vi "HEWH Find Draw Start.vi"(6 "Loop Index":i32, 7 "Index Type":T1, 8 "Error In":errorcluster, 10 "Start Index":i32, 11 "UEF Calculated Values in":T2 {"Data Indexes"."15 sec after Draw Index" format="%#.2f"; "Data Indexes"."15 sec after Draw Timestamp" format="%#.2f"; "Data Indexes"."Test Start Timestamp" format="%.2f"; "Data Indexes"."Test End Timestamp" format="%.2f"; "Data Indexes"."T0 Timestamp" format="%.2f"; "Data Indexes"."Tsf Timestamp" format="%.2f"; "Data Indexes"."Tsu0 Timestamp" format="%.2f"; "Data Indexes"."Tmax1 Timestamp" format="%.2f"; "Data Indexes"."Draw Index Timestamp" format="%#.2f"; "Data Indexes"."Non-Draw Timestamp" format="%#.2f"; "Data Indexes"."Heating Timestamp" format="%#.2f"; "Data Indexes"."Start Energy (BTU-Gas)" format="%.6f"; "Data Indexes"."Start Watt Hours" format="%.6f"; "Static Data"."V - Volume of Wh (True)" format="%.5f"; "Static Data"."T-Ambinet Nominal (°F)" format="%.5f"; "Static Data"."T-Inlet Setpoint (°F)" format="%.5f"; "Static Data"."T-Wh Setpoint (°F)" format="%.5f"; "Sampled Data"."Qe (Wh)" format="%.5f"; "Sampled Data"."Tau stby2 (hr)" format="%.5f"; "Sampled Data"."Tastby2 (°F)" format="%.5f"; "Sampled Data"."Qf (BTU)" format="%.5f"; "Sampled Data"."Qe (BTU)" format="%.5f"; "Sampled Data"."Tmax1 (°F)" format="%.5f"; "Sampled Data"."T0 (°F)" format="%.5f"; "Sampled Data"."Qr (BTU)" format="%.5f"; "Sampled Data"."T 24(°F)" format="%.5f"; "Sampled Data"."T astby(°F)" format="%.5f"; "Sampled Data"."T tstby(°F)" format="%.5f"; "Sampled Data"."T su0(°F)" format="%.5f"; "Sampled Data"."T suf(°F)" format="%.5f"; "Sampled Data"."Tau stby_1 (hr)" format="%.5f"; "Sampled Data"."Qsuf (BTU)" format="%.5f"; "Sampled Data"."Qsu0 (BTU)" format="%.5f"; "Calculated Values"."Draw Bonus Volume (gal)" format="%.6f"; "Calculated Values"."Adjustment Factor" format="%.6f"; "Calculated Values"."T*avg_del(n-1)" format="%.6f"; "Calculated Values"."T*min(n-1)" format="%.6f"; "Calculated Values"."T*avg_del(n)" format="%.6f"; "Calculated Values"."Vn" format="%.6f"; "Calculated Values"."Qdm (BTU)" format="%.6f"; "Calculated Values"."QHWD (BTU)" format="%.6f"; "Calculated Values"."QHW (BTU)" format="%.6f"; "Calculated Values"."UEF" format="%.6f"; "Calculated Values"."QHW67 (BTU)" format="%.6f"; "Calculated Values"."Qda (BTU)" format="%.6f"; "Calculated Values"."Qd (BTU)" format="%.6f"; "Calculated Values"."Q (BTU)" format="%.6f"; "Calculated Values"."UA (BTU/(hr*F))" format="%.6f"; "Calculated Values"."Qhr (BTU/hr)" format="%.6f"; "Calculated Values"."Qstby (BTU)" format="%.6f"; "Calculated Values"."nu_r" format="%.6f"; "Calculated Values"."CpUEF (BTU/(lb*F))" format="%.6f"; "Calculated Values"."rho_nu (lb/gal)" format="%.6f"; "Calculated Values"."V1- Vol (Gal)" format="%.6f"; "Calculated Values"."M cluster mass removed (lb)" format="%.6f"; "Calculated Values"."Cp theoretical (BTU/(lbm °F))" format="%.6f"; "Calculated Values"."Tin1 - Mean Inlet 1st Cluster (°F)" format="%.6f"; "Calculated Values"."Tdel1-Mean Outlet 1st Cluster(°F)" format="%.6f"; "Calculated Values"."Cp 24 (BTU/(lb*F))" format="%.6f"; "Calculated Values"."Cp standby (BTU/(lb*F))" format="%.6f"; "Calculated Values"."Cp2 (BTU/(lb*F))" format="%.6f"; "Calculated Values"."Cp1 (BTU/(lb*F))" format="%.6f"; "Calculated Values"."rho 24 (lb/gal)" format="%.6f"; "Calculated Values"."rho standby (lb/gal)" format="%.6f"; "Calculated Values"."rho 2 (lb/gal)" format="%.6f"; "Calculated Values"."Density of cold water All (lbm/gal)" format="%#.3g"; "Calculated Values"."CpHW (BTU/(lbm °F))" format="%#.3g"; "Calculated Values"."Density of hot water All (lbm/gal)" format="%#.3g"; "Calculated Values"."Mass of water All (lbm)" format="%#.3f"}) -> (0 "Error Out":errorcluster, 1 "Stop Searching":bool, 2 "Draw Start":i32, 3 "UEF Calculated Values Output":T2 {"Data Indexes"."15 sec after Draw Index" format="%#.2f"; "Data Indexes"."15 sec after Draw Timestamp" format="%#.2f"; "Data Indexes"."Test Start Timestamp" format="%.2f"; "Data Indexes"."Test End Timestamp" format="%.2f"; "Data Indexes"."T0 Timestamp" format="%.2f"; "Data Indexes"."Tsf Timestamp" format="%.2f"; "Data Indexes"."Tsu0 Timestamp" format="%.2f"; "Data Indexes"."Tmax1 Timestamp" format="%.2f"; "Data Indexes"."Draw Index Timestamp" format="%#.2f"; "Data Indexes"."Non-Draw Timestamp" format="%#.2f"; "Data Indexes"."Heating Timestamp" format="%#.2f"; "Data Indexes"."Start Energy (BTU-Gas)" format="%.6f"; "Data Indexes"."Start Watt Hours" format="%.6f"; "Static Data"."V - Volume of Wh (True)" format="%.5f"; "Static Data"."T-Ambinet Nominal (°F)" format="%.5f"; "Static Data"."T-Inlet Setpoint (°F)" format="%.5f"; "Static Data"."T-Wh Setpoint (°F)" format="%.5f"; "Sampled Data"."Qe (Wh)" format="%.5f"; "Sampled Data"."Tau stby2 (hr)" format="%.5f"; "Sampled Data"."Tastby2 (°F)" format="%.5f"; "Sampled Data"."Qf (BTU)" format="%.5f"; "Sampled Data"."Qe (BTU)" format="%.5f"; "Sampled Data"."Tmax1 (°F)" format="%.5f"; "Sampled Data"."T0 (°F)" format="%.5f"; "Sampled Data"."Qr (BTU)" format="%.5f"; "Sampled Data"."T 24(°F)" format="%.5f"; "Sampled Data"."T astby(°F)" format="%.5f"; "Sampled Data"."T tstby(°F)" format="%.5f"; "Sampled Data"."T su0(°F)" format="%.5f"; "Sampled Data"."T suf(°F)" format="%.5f"; "Sampled Data"."Tau stby_1 (hr)" format="%.5f"; "Sampled Data"."Qsuf (BTU)" format="%.5f"; "Sampled Data"."Qsu0 (BTU)" format="%.5f"; "Calculated Values"."Draw Bonus Volume (gal)" format="%.6f"; "Calculated Values"."Adjustment Factor" format="%.6f"; "Calculated Values"."T*avg_del(n-1)" format="%.6f"; "Calculated Values"."T*min(n-1)" format="%.6f"; "Calculated Values"."T*avg_del(n)" format="%.6f"; "Calculated Values"."Vn" format="%.6f"; "Calculated Values"."Qdm (BTU)" format="%.6f"; "Calculated Values"."QHWD (BTU)" format="%.6f"; "Calculated Values"."QHW (BTU)" format="%.6f"; "Calculated Values"."UEF" format="%.6f"; "Calculated Values"."QHW67 (BTU)" format="%.6f"; "Calculated Values"."Qda (BTU)" format="%.6f"; "Calculated Values"."Qd (BTU)" format="%.6f"; "Calculated Values"."Q (BTU)" format="%.6f"; "Calculated Values"."UA (BTU/(hr*F))" format="%.6f"; "Calculated Values"."Qhr (BTU/hr)" format="%.6f"; "Calculated Values"."Qstby (BTU)" format="%.6f"; "Calculated Values"."nu_r" format="%.6f"; "Calculated Values"."CpUEF (BTU/(lb*F))" format="%.6f"; "Calculated Values"."rho_nu (lb/gal)" format="%.6f"; "Calculated Values"."V1- Vol (Gal)" format="%.6f"; "Calculated Values"."M cluster mass removed (lb)" format="%.6f"; "Calculated Values"."Cp theoretical (BTU/(lbm °F))" format="%.6f"; "Calculated Values"."Tin1 - Mean Inlet 1st Cluster (°F)" format="%.6f"; "Calculated Values"."Tdel1-Mean Outlet 1st Cluster(°F)" format="%.6f"; "Calculated Values"."Cp 24 (BTU/(lb*F))" format="%.6f"; "Calculated Values"."Cp standby (BTU/(lb*F))" format="%.6f"; "Calculated Values"."Cp2 (BTU/(lb*F))" format="%.6f"; "Calculated Values"."Cp1 (BTU/(lb*F))" format="%.6f"; "Calculated Values"."rho 24 (lb/gal)" format="%.6f"; "Calculated Values"."rho standby (lb/gal)" format="%.6f"; "Calculated Values"."rho 2 (lb/gal)" format="%.6f"; "Calculated Values"."Density of cold water All (lbm/gal)" format="%#.3g"; "Calculated Values"."CpHW (BTU/(lbm °F))" format="%#.3g"; "Calculated Values"."Density of hot water All (lbm/gal)" format="%#.3g"; "Calculated Values"."Mass of water All (lbm)" format="%#.3f"})   [LabVIEW 2023]
uses:
  Type Definitions/UEF Constants.ctl
  Type Definitions/HEWH Draw Stats.ctl
  Type Definitions/HEWH FHR Draw Type.ctl
  Type Definitions/FHR Bins.ctl
  Type Definitions/HEWH Meter Type.ctl
  Type Definitions/HEWH Index Type.ctl
panel:
  out "Raw Data.Test Data-Start to End DBL":dbl[][](array[numeric])
  # "FHR"
  # "FHR"
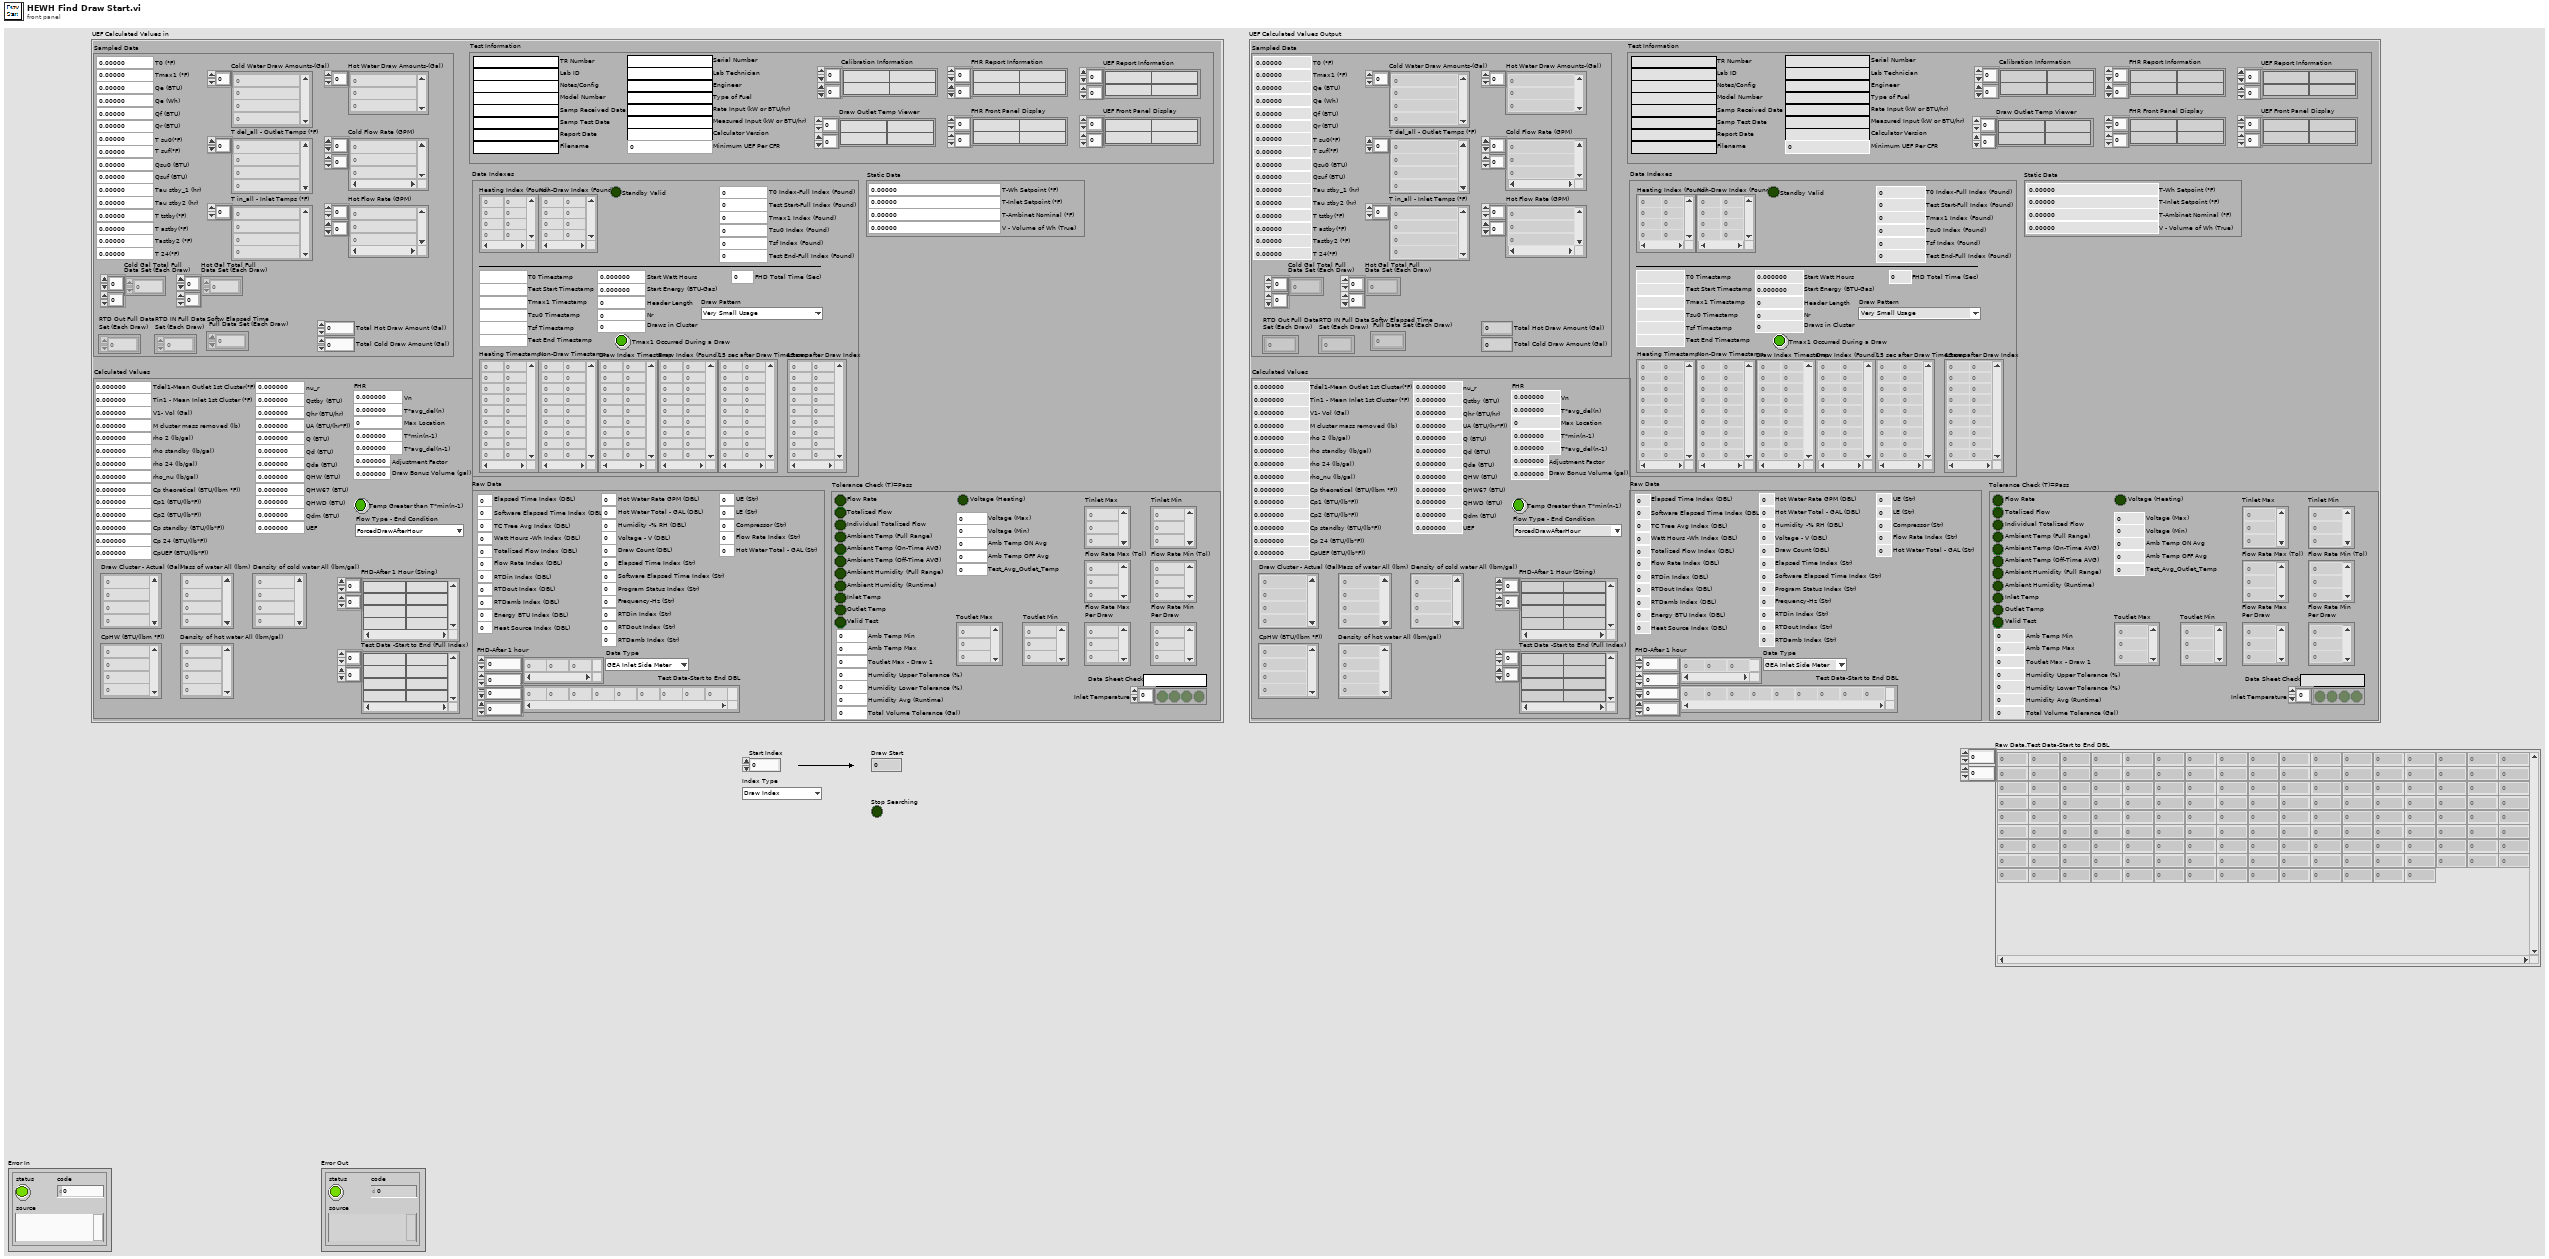
[diagram p1: front panel]
types:
  T1 = typedef "HEWH Index Type.ctl" = enum16{"Draw Index", "Heating Index", "Temp Based (FHD)"}
  T2 = typedef "UEF Constants.ctl" = cluster{"Calculated Values":T3, "Sampled Data":cluster{"Cold Water Draw Amounts-(Gal)":dbl[], "T del_all - Outlet Temps (°F)":dbl[], "T in_all - Inlet Temps (°F)":dbl[], "Qsu0 (BTU)":dbl, "Qsuf (BTU)":dbl, "Tau stby_1 (hr)":dbl, "T suf(°F)":dbl, "T su0(°F)":dbl, "T tstby(°F)":dbl, "T astby(°F)":dbl, "T 24(°F)":dbl, "Qr (BTU)":dbl, "T0 (°F)":dbl, "Tmax1 (°F)":dbl, "Qe (BTU)":dbl, "Qf (BTU)":dbl, "Tastby2 (°F)":dbl, "RTD Out Full Data\nSet (Each Draw)":dbl[][], "RTD IN Full Data\nSet (Each Draw)":dbl[][], "Tau stby2 (hr)":dbl, "Hot Water Draw Amounts-(Gal)":dbl[], "Cold Flow Rate (GPM)":dbl[][], "Hot Flow Rate (GPM)":dbl[][], "Softw Elapsed Time\n Full Data Set (Each Draw)":dbl[][], "Cold Gal Total Full\nData Set (Each Draw)":dbl[][], "Total Hot Draw Amount (Gal) ":dbl, "Total Cold Draw Amount (Gal)":dbl, "Qe (Wh)":dbl, "Hot Gal Total Full\nData Set (Each Draw)":dbl[][]}, "Static Data":cluster{"T-Wh Setpoint (°F)":dbl, "T-Inlet Setpoint (°F)":dbl, "T-Ambinet Nominal (°F)":dbl, "V - Volume of Wh (True)":dbl}, "Data Indexes":cluster{"Test Start-Full Index (Found)":i32, "Header Length":i32, "Draw Index (Found)":i32[][], "Nr":i32, "Start Watt Hours":dbl, "Tsu0 Index (Found)":i32, "Tsf Index (Found)":i32, "Start Energy (BTU-Gas)":dbl, "Draws in Cluster":i32, "T0 Index-Full Index (Found)":i32, "Non-Draw Index (Found)":i32[][], "Tmax1 Index (Found)":i32, "Test End-Full Index (Found)":i32, "Heating Index (Found)":i32[][], "Heating Timestamp":dbl[][], "Non-Draw Timestamp":dbl[][], "Draw Index Timestamp":dbl[][], "Tmax1 Timestamp":dbl, "Tsu0 Timestamp":dbl, "Tsf Timestamp":dbl, "T0 Timestamp":dbl, "Test End Timestamp":dbl, "Test Start Timestamp":dbl, "15 sec after Draw Timestamp":dbl[][], "15 sec after Draw Index":dbl[][], "Tmax1 Occurred During a Draw":bool, "FHD Total Time (Sec)":dbl, "Draw Pattern":T5, "Standby Valid":bool}, "Raw Data":cluster{"Elapsed Time Index (DBL)":i32, "Software Elapsed Time Index (DBL)":i32, "TC Tree Avg Index (DBL)":i32, "Watt Hours -Wh Index (DBL)":i32, "Energy BTU Index (DBL)":i32, "Totalized Flow Index (DBL)":i32, "Flow Rate Index (DBL)":i32, "Program Status Index (Str)":i32, "RTDin Index (DBL)":i32, "RTDout Index (DBL)":i32, "RTDamb Index (DBL)":i32, "Test Data-Start to End DBL":dbl[][], "Data Type":T6, "Heat Source Index (DBL)":i32, "Hot Water Rate GPM (DBL)":i32, "Hot Water Total - GAL (DBL)":i32, "FHD-After 1 hour":dbl[][], "Humidity -% RH (DBL)":i32, "Voltage - V (DBL)":i32, "Draw Count (DBL)":i32, "Elapsed Time Index (Str)":i32, "Software Elapsed Time Index (Str)":i32, "Frequency-Hz (Str)":i32, "RTDin Index (Str)":i32, "RTDout Index (Str)":i32, "RTDamb Index (Str)":i32, "UE (Str)":i32, "LE (Str)":i32, "Compressor (Str)":i32, "Flow Rate Index (Str)":i32, "Hot Water Total - GAL (Str)":i32}, "Tolerance Check (T)=Pass":cluster{"Flow Rate":bool, "Totalized Flow":bool, "Ambient Temp (Full Range)":bool, "Ambient Humidity (Full Range)":bool, "Inlet Temp":bool, "Outlet Temp":bool, "Valid Test":bool, "Individual Totalized Flow":bool, "Data Sheet Check":string, "Inlet Temperature":bool[], "Tinlet Max":dbl[], "Tinlet Min":dbl[], "Flow Rate Max (Tol)":dbl[], "Flow Rate Min (Tol)":dbl[], "Amb Temp Max":dbl, "Amb Temp Min":dbl, "Toutlet Max - Draw 1":dbl, "Humidity Upper Tolerance (%)":dbl, "Total Volume Tolerance (Gal)":dbl, "Humidity Lower Tolerance (%)":dbl, "Flow Rate Max\nPer Draw":dbl[], "Flow Rate Min\nPer Draw":dbl[], "Ambient Humidity (Runtime)":bool, "Humidity Avg (Runtime)":dbl, "Ambient Temp (On-Time AVG)":bool, "Ambient Temp (Off-Time AVG)":bool, "Amb Temp OFF Avg":dbl, "Amb Temp ON Avg":dbl, "Voltage (Heating)":bool, "Voltage (Min)":dbl, "Voltage (Max)":dbl, "Toutlet Max":dbl[], "Toutlet Min":dbl[], "Test_Avg_Outlet_Temp":dbl}, "Test Information":cluster{"TR Number":string, "Lab ID":string, "Notes/Config":string, "Model Number":string, "Serial Number":string, "Lab Technician":string, "Engineer":string, "Type of Fuel":string, "Samp Received Date":string, "Samp Test Date":string, "Report Date":string, "Rate Input (kW or BTU/hr)":string, "Measured Input (kW or BTU/hr)":string, "Filename":string, "Calibration Information":string[][], "Calculator Version":string, "Minimum UEF Per CFR":dbl, "UEF Report Information":string[][], "FHR Report Information":string[][], "FHR Front Panel Display":string[][], "UEF Front Panel Display":string[][], "Draw Outlet Temp Viewer":string[][]}}
  T3 = typedef "HEWH Draw Stats.ctl" = cluster{"Draw Cluster - Actual (Gal)":dbl[], "Mass of water All (lbm)":dbl[], "Density of hot water All (lbm/gal)":dbl[], "CpHW (BTU/(lbm °F))":dbl[], "rho 2 (lb/gal)":dbl, "rho standby (lb/gal)":dbl, "rho 24 (lb/gal)":dbl, "Cp1 (BTU/(lb*F))":dbl, "Cp2 (BTU/(lb*F))":dbl, "Cp standby (BTU/(lb*F))":dbl, "Cp 24 (BTU/(lb*F))":dbl, "nu_r":dbl, "Qstby (BTU)":dbl, "Qhr (BTU/hr)":dbl, "UA (BTU/(hr*F))":dbl, "Q (BTU)":dbl, "Qd (BTU)":dbl, "Qda (BTU)":dbl, "QHW67 (BTU)":dbl, "UEF":dbl, "Tdel1-Mean Outlet 1st Cluster(°F)":dbl, "Tin1 - Mean Inlet 1st Cluster (°F)":dbl, "Cp theoretical (BTU/(lbm °F))":dbl, "M cluster mass removed (lb)":dbl, "V1- Vol (Gal)":dbl, "Test Data -Start to End (Full Index)":string[][], "rho_nu (lb/gal)":dbl, "Density of cold water All (lbm/gal)":dbl[], "CpUEF (BTU/(lb*F))":dbl, "QHW (BTU)":dbl, "QHWD (BTU)":dbl, "Qdm (BTU)":dbl, "FHD-After 1 Hour (String)":string[][], "Vn":dbl, "T*avg_del(n)":dbl, "Max Location":i32, "T*min(n-1)":dbl, "T*avg_del(n-1)":dbl, "Temp Greater than T*min(n-1)":bool, "Adjustment Factor":dbl, "Draw Bonus Volume (gal)":dbl, "Flow Type - End Condition":T4}
  T4 = typedef "HEWH FHR Draw Type.ctl" = enum16{"ForcedDrawAfterHour", "HeatingCutoffBeforeHour"}
  T5 = typedef "FHR Bins.ctl" = enum16{"Very Small Usage", "Low Usage", "Medium Usage", "High Usage", "Undefined"}
  T6 = typedef "HEWH Meter Type.ctl" = enum16{"GEA Inlet Side Meter", "GEA Outlet Side Meter", "CSA Inlet Side Meter"}
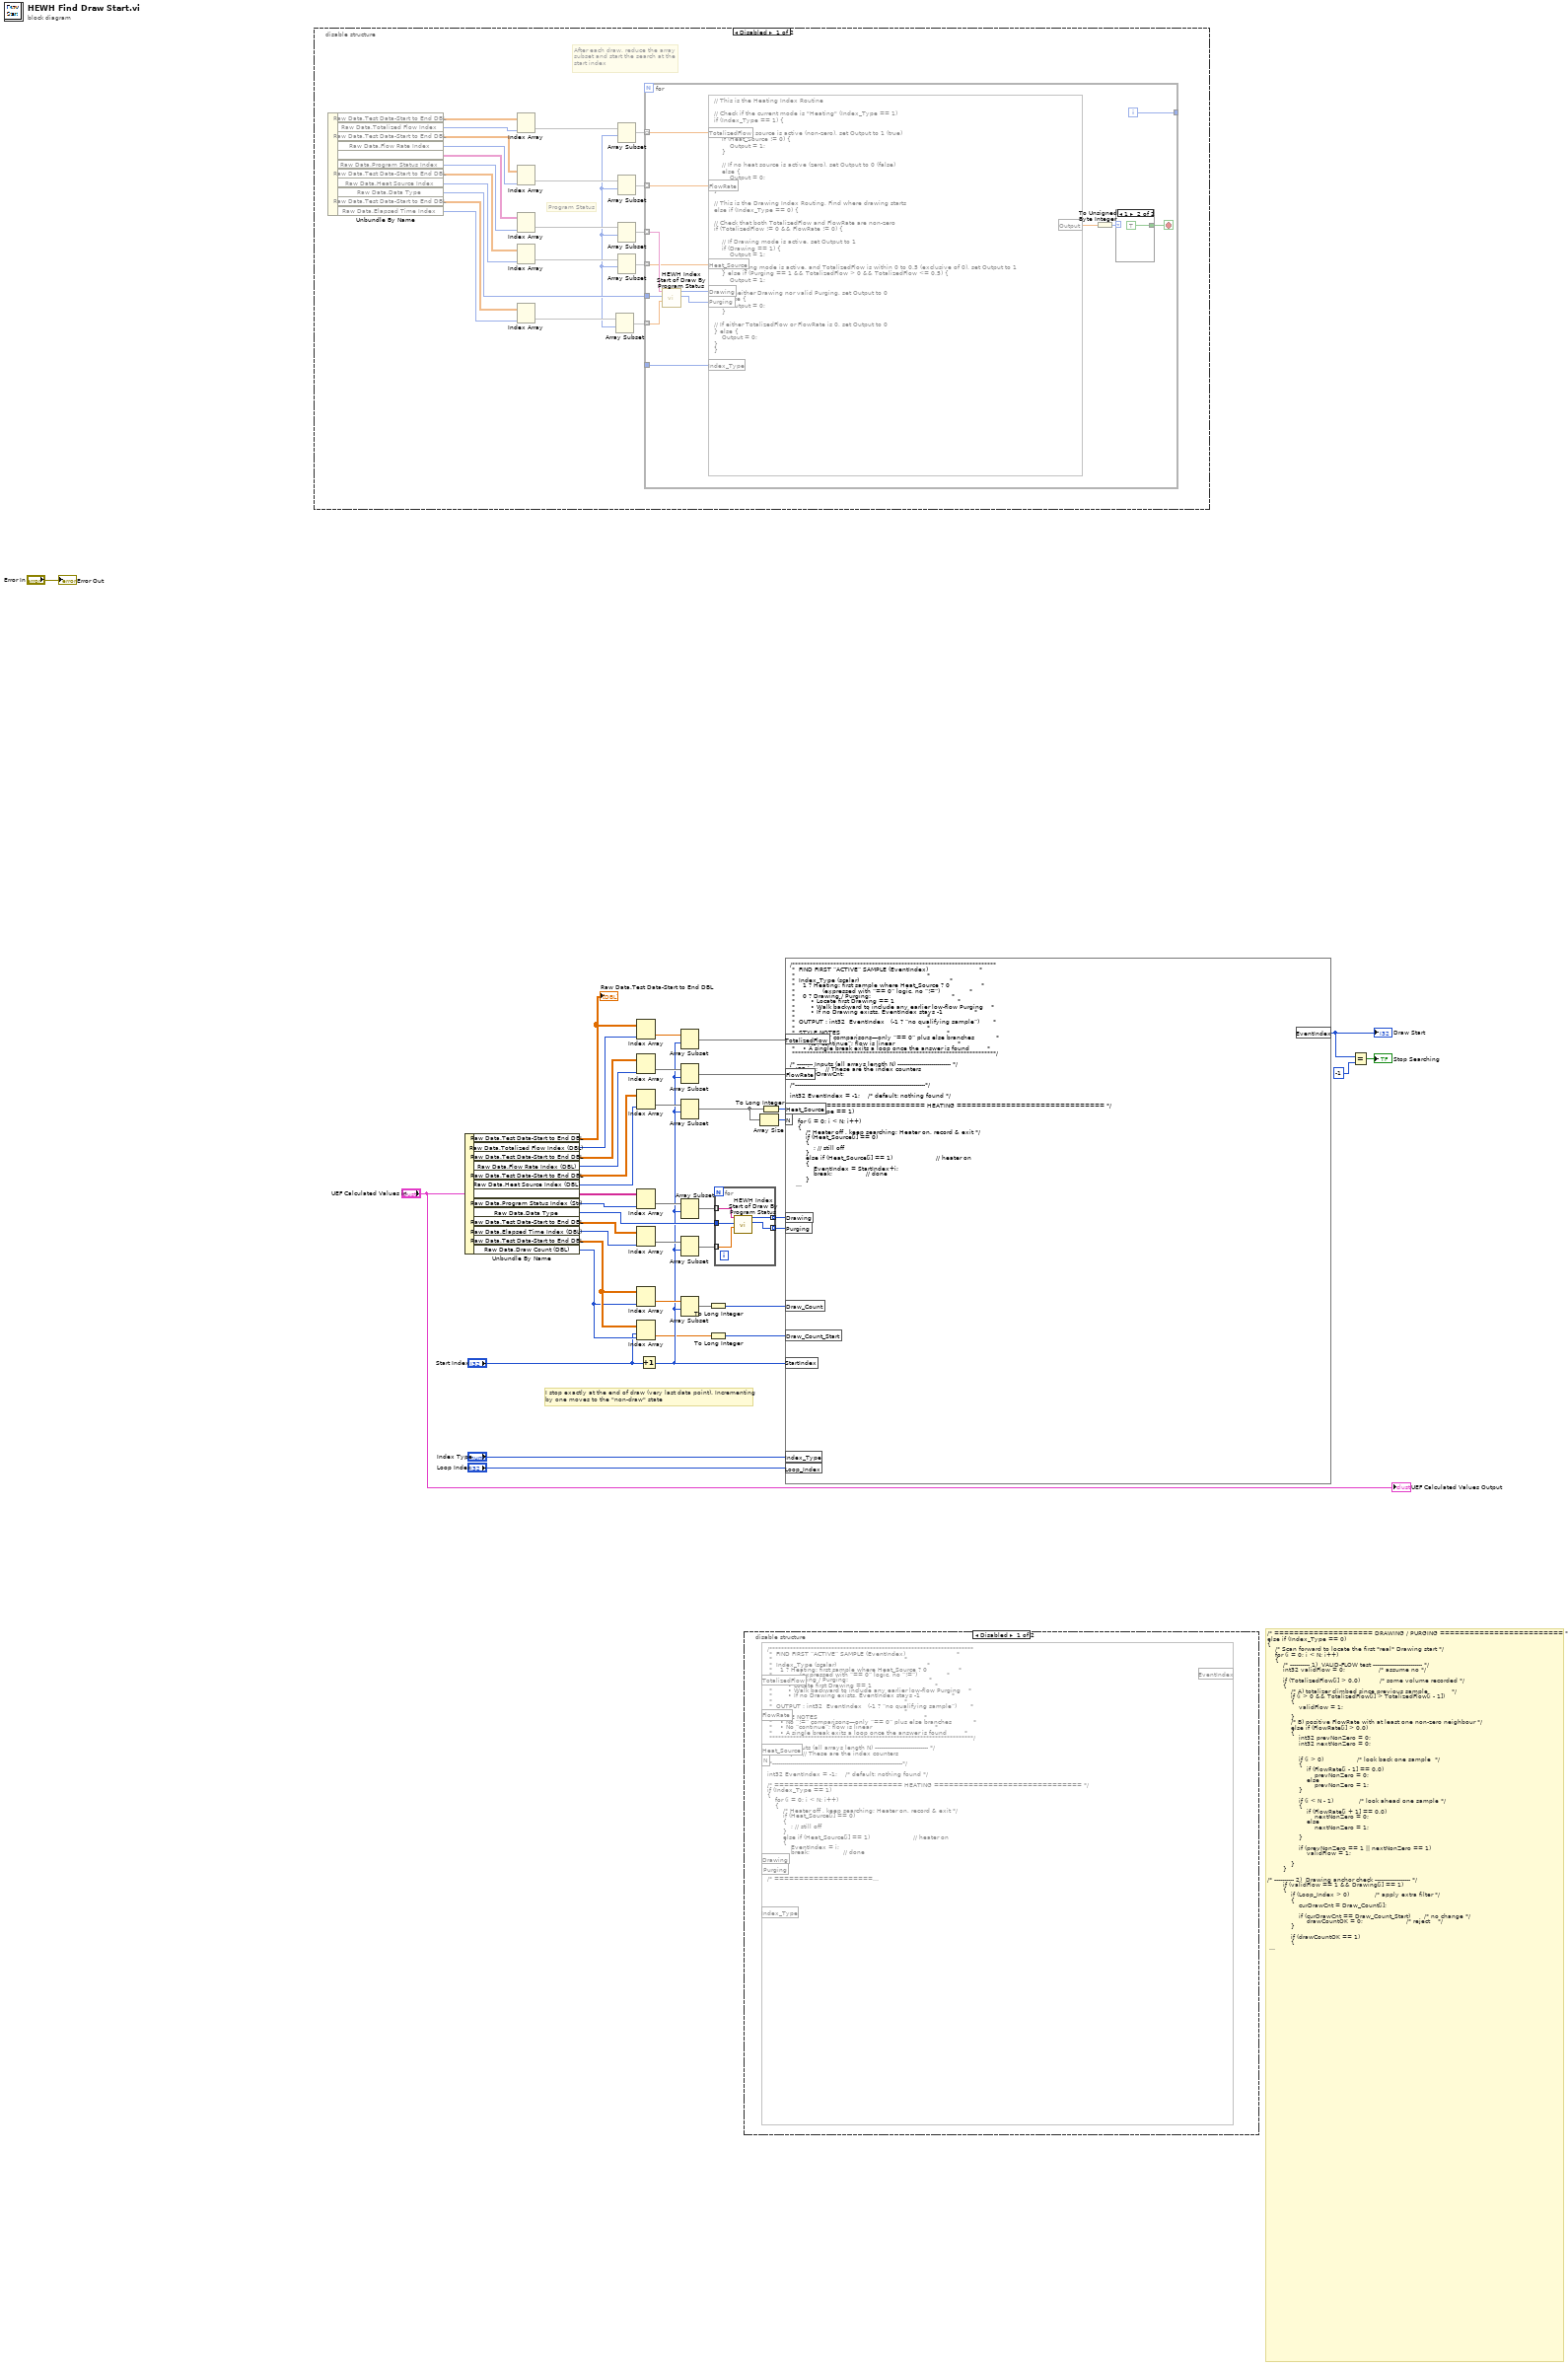
[diagram p0: block diagram]
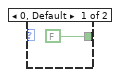
[diagram p3: hidden frame]
diagram:
  # "/* ==================== DRAWING / PURGING ========================= */\nelse if (Index_Type == 0)\n{\n    /* Scan forward to locate the first *real* Drawing start */\n    for (i = 0; i < N; i++)\n    {\n        /* ---------- 1)  VALID-FLOW test ------------------------- */\n        int32 validFlow = 0;                 /* assume no */\n\n        if (TotalizedFlow[i] > 0.0)          /* some volume recorded */\n        {\n            /* A) totalizer climbed since previous sample            */\n            if (i > 0 && TotalizedFlow[i] > TotalizedFlow[i - 1])\n            {\n                validFlow = 1;\n                \n            }\n            /* B) positive FlowRate with at least one non-zero neighbour */\n            else if (FlowRate[i] > 0.0)\n            {\n                int32 prevNonZero = 0;\n                int32 nextNonZero = 0;\n                \n\n                if (i > 0)                 /* look back one sample  */\n                {\n                    if (FlowRate[i - 1] == 0.0)\n                        prevNonZero = 0;\n                    else\n                        prevNonZero = 1;\n                }\n\n                if (i < N - 1)             /* look ahead one sample */\n                {\n                    if (FlowRate[i + 1] == 0.0)\n                        nextNonZero = 0;\n                    else\n                        nextNonZero = 1;\n                        \n                }\n\n                if (prevNonZero == 1 || nextNonZero == 1)\n                    validFlow = 1;\n                    \n            }\n        }\n\n/* ---------- 2)  Drawing anchor check ------------------ */\n        if (validFlow == 1 && Drawing[i] == 1)\n        {\n            if (Loop_Index > 0)             /* apply extra filter */\n            {\n                curDrawCnt = Draw_Count[i];\n\n                if (curDrawCnt == Draw_Count_Start)       /* no change */\n                    drawCountOK = 0;                      /* reject    */\n            }\n\n            if (drawCountOK == 1)\n            {\n                EventIndex = StartIndex + i;              /* anchor    */\n\n                /* ---- back-fill earlier low-flow Purging ------ */\n                for (j = i - 1; j >= 0; j--)\n                {\n                    if (Purging[j] == 1 &&\n                        TotalizedFlow[j] > 0.0 &&\n                        TotalizedFlow[j] <= 0.5)\n                    {\n                        EventIndex = StartIndex + j;      /* shift back */\n                    }\n                    else\n                    {\n                        break;                            /* leave zone */\n                    }\n                }\n                break;                                   /* anchor done */\n            }\n        }\n        /* else: keep scanning */\n    }\n}\n/* ===== any other Index_Type – EventIndex remains -1 ============ */"
  # "I stop exactly at the end of draw (very last data point). Incrementing\nby one moves to the \"non-draw\" state"
  n1 = disable-structure shown="Disabled" {
    frame Disabled {
      # "Program Status"
      # "After each draw, reduce the array\nsubset and start the search at the \nstart index"
      n2 = Unbundle By Name() -> ("Raw Data.Test Data-Start to End DBL"=w60:dbl[][], "Raw Data.Totalized Flow Index"=w63:i32, "Raw Data.Test Data-Start to End DBL"=w47:dbl[][], "Raw Data.Flow Rate Index"=w62:i32, "Calculated Values.Test Data -Start to End (Full Index)"=w59:string[][], "Raw Data.Program Status Index"=w61:i32, "Raw Data.Test Data-Start to End DBL"=w53:dbl[][], "Raw Data.Heat Source Index"=w52:i32, "Raw Data.Data Type"=w49:T6, "Raw Data.Test Data-Start to End DBL"=w46:dbl[][], "Raw Data.Elapsed Time Index"=w45:i32)  [unwired: 1 in]
      n3 = Index Array(array=w60, index (col)=w63) -> (element=w48:dbl[])  [unwired: 1 in]
      n4 = Index Array(array=w47, index (col)=w62) -> (element=w58:dbl[])  [unwired: 1 in]
      n5 = Index Array(array=w59, index (col)=w61) -> (element=w57:string[])  [unwired: 1 in]
      n6 = Index Array(array=w53, index (col)=w52) -> (element=w51:dbl[])  [unwired: 1 in]
      n7 = Index Array(array=w46, index (col)=w45) -> (element=w44:dbl[])  [unwired: 1 in]
      n8 = Array Subset(array=w58) -> (w55:dbl[], index=w42:i32)  [unwired: 1 in]
      n9 = Array Subset(array=w44, index=w42) -> (w43:dbl[])  [unwired: 1 in]
      n10 = Array Subset(array=w48, index=w42) -> (w54:dbl[])  [unwired: 1 in]
      n11 = Array Subset(array=w57, index=w42) -> (w56:string[])  [unwired: 1 in]
      n12 = Array Subset(array=w51, index=w42) -> (w50:dbl[])  [unwired: 1 in]
      n13 = for {
        tunnel: w56 -> [w72] mode=indexing
        tunnel: [w76] -> _
        tunnel: w54 -> [w75] mode=indexing
        tunnel: w55 -> [w74] mode=indexing
        tunnel: w50 -> [w71] mode=indexing
        tunnel: w49 -> [w70]
        tunnel: _ -> [w69]
        tunnel: w43 -> [w64] mode=indexing
        i -> [w76]
        stop <- w73 stop-if-true
        n14 = call "HEWH Index Start of Draw By Program Status.vi"("Elapsed Time (sec)"=w64, "Data Type"=w70, "Program Status"=w72) -> ("Purging"=w66:i16, "Drawing"=w65:i16)  [unwired: 7 in]
        n15 = formula code="// This is the Heating Index Routine\n\n// Check if the current mode is \"Heating\" (Index_Type == 1)\nif (Index_Type == 1) {\n\n    // If a heat source is active (non-zero), set Output to 1 (true)\n    if (Heat_Source != 0) {\n        Output = 1;\n    } \n    \n    // If no heat source is active (zero), set Output to 0 (false)\n    else {\n        Output = 0;\n    }\n}\n\n// This is the Drawing Index Routing, Find where drawing starts\nelse if (Index_Type == 0) {\n\n// Check that both TotalizedFlow and FlowRate are non-zero\nif (TotalizedFlow != 0 && FlowRate != 0) {\n\n    // If Drawing mode is active, set Output to 1\n    if (Drawing == 1) {\n        Output = 1;\n\n    // If Purging mode is active, and TotalizedFlow is within 0 to 0.5 (exclusive of 0), set Output to 1\n    } else if (Purging == 1 && TotalizedFlow > 0 && TotalizedFlow <= 0.5) {\n        Output = 1;\n\n    // If neither Drawing nor valid Purging, set Output to 0\n    } else {\n        Output = 0;\n    }\n\n// If either TotalizedFlow or FlowRate is 0, set Output to 0\n} else {\n    Output = 0;\n}\n}"("TotalizedFlow"=w75, "FlowRate"=w74, "Drawing"=w65, "Purging"=w66, "Index_Type"=w69, "Heat_Source"=w71) -> ("Output"=w67:dbl)
        n16 = To Unsigned Byte Integer(number=w67) -> (unsigned 8bit integer=w68:u8)
        n17 = case shown="1" w68 {
          tunnel: [FALSE TRUE] -> w73
          frame 0, Default {
          }
          frame 1 {
          }
        }
      }
    }
    frame Enabled {
    }
  }
  n18 = Unbundle By Name("UEF Calculated Values in") -> ("Raw Data.Test Data-Start to End DBL"=w26:dbl[][], "Raw Data.Totalized Flow Index (DBL)"=w25:i32, "Raw Data.Test Data-Start to End DBL"=w23:dbl[][], "Raw Data.Flow Rate Index (DBL)"=w22:i32, "Raw Data.Test Data-Start to End DBL"=w19:dbl[][], "Raw Data.Heat Source Index (DBL)"=w18:i32, "Calculated Values.Test Data -Start to End (Full Index)"=w36:string[][], "Raw Data.Program Status Index (Str)"=w35:i32, "Raw Data.Data Type"=w32:T6, "Raw Data.Test Data-Start to End DBL"=w39:dbl[][], "Raw Data.Elapsed Time Index (DBL)"=w38:i32, "Raw Data.Test Data-Start to End DBL"=w5:dbl[][], "Raw Data.Draw Count (DBL)"=w4:i32)
  "Raw Data.Test Data-Start to End DBL" <- w26
  n19 = Index Array(array=w26, index (col)=w25) -> (element=w27:dbl[])  [unwired: 1 in]
  n20 = Index Array(array=w23, index (col)=w22) -> (element=w21:dbl[])  [unwired: 1 in]
  n21 = Index Array(array=w19, index (col)=w18) -> (element=w13:dbl[])  [unwired: 1 in]
  n22 = Index Array(array=w36, index (col)=w35) -> (element=w34:string[])  [unwired: 1 in]
  n23 = Index Array(array=w39, index (col)=w38) -> (element=w37:dbl[])  [unwired: 1 in]
  n24 = Index Array(array=w5, index (col)=w4) -> (element=w9:dbl[])  [unwired: 1 in]
  n25 = Index Array(array=w5, index (row)="Start Index", index (col)=w4) -> (element=w2:dbl)
  n26 = Increment(x="Start Index") -> (x+1=w8:i32)
  n27 = Array Subset(array=w27, index=w8) -> (w24:dbl[])  [unwired: 1 in]
  n28 = Array Subset(array=w21, index=w8) -> (w20:dbl[])  [unwired: 1 in]
  n29 = Array Subset(array=w13, index=w8) -> (w12:dbl[])  [unwired: 1 in]
  n30 = Array Subset(array=w34, index=w8) -> (w31:string[])  [unwired: 1 in]
  n31 = Array Subset(array=w37, index=w8) -> (w33:dbl[])  [unwired: 1 in]
  n32 = Array Subset(array=w9, index=w8) -> (w7:dbl[])  [unwired: 1 in]
  n33 = To Long Integer(number=w7) -> (32bit integer=w6:i32[])
  n34 = To Long Integer(number=w2) -> (32bit integer=w1:i32)
  n35 = for {
    tunnel: w33 -> [w83] mode=indexing
    tunnel: w32 -> [w82]
    tunnel: w31 -> [w81] mode=indexing
    tunnel: [w80] -> w29 mode=indexing
    tunnel: [w79] -> w30 mode=indexing
    n36 = call "HEWH Index Start of Draw By Program Status.vi"("Elapsed Time (sec)"=w83, "Data Type"=w82, "Program Status"=w81) -> ("Purging"=w79:i16, "Drawing"=w80:i16)  [unwired: 7 in]
  }
  n37 = disable-structure shown="Disabled" {
    frame Disabled {
      # "/* ---------- 2)  Drawing anchor check -------------------- */\n        if (validFlow == 1 && Drawing[i] == 1 && Test_Data_StartToEnd[StartIndex+i][DrawCountIndex] !=Draw_Count_Start)\n        {\n            EventIndex = StartIndex+i;                 /* provisional anchor */                \n\n            /* -------- back-fill earlier low-flow Purging -------- */\n            for (j = i - 1; j >= 0; j--)\n            {\n                if (Purging[j] == 1 &&\n                    TotalizedFlow[j] > 0.0 &&\n                    TotalizedFlow[j] <= 0.5)\n                {\n                    EventIndex = StartIndex+j;         /* shift anchor back */\n                }\n                else\n                {\n                    break;                  /* left back-fill zone */\n                }\n            }\n            break;                          /* anchor secured; stop */\n        }\n        /* else: keep looping to next i */\n    }\n}\n/* ===== any other Index_Type – EventIndex remains -1 ============ */"
      n38 = formula code="/*********************************************************************\n *  FIND FIRST “ACTIVE” SAMPLE (EventIndex)                          *\n *                                                                   *\n *  Index_Type (scalar)                                              *\n *    1 ? Heating: first sample where Heat_Source ? 0                *\n *              (expressed with “== 0” logic, no “!=”)               *\n *    0 ? Drawing / Purging:                                         *\n *        • Locate first Drawing == 1                                *\n *        • Walk backward to include any earlier low-flow Purging    *\n *        • If no Drawing exists, EventIndex stays -1                *\n *                                                                   *\n *  OUTPUT : int32  EventIndex   (-1 ? “no qualifying sample”)       *\n *                                                                   *\n *  STYLE NOTES                                                      *\n *    • No “!=” comparisons—only “== 0” plus else branches           *\n *    • No “continue”; flow is linear                                *\n *    • A single break exits a loop once the answer is found         *\n *********************************************************************/\n\n/* -------- Inputs (all arrays length N) --------------------------- */\nint32 i, j;    // These are the index counters\n\n/*------------------------------------------------------------------*/\n\nint32 EventIndex = -1;    /* default: nothing found */\n\n/* ========================== HEATING ============================== */\nif (Index_Type == 1)\n{\n    for (i = 0; i < N; i++)\n    {\n        /* Heater off , keep searching; Heater on, record & exit */\n        if (Heat_Source[i] == 0)\n        {\n            ; // still off\n        }\n        else if (Heat_Source[i] == 1)                      // heater on\n        {\n            EventIndex = i;\n            break;                 // done\n        }\n    }\n}\n\n/* ==================== DRAWING / PURGING ========================= */\nelse if (Index_Type == 0)\n{\n    /* PASS: look for first Drawing == 1 and back-fill purging */\n    for (i = 0; i < N; i++)\n    {\n        /* skip samples with no flow */\n        if (TotalizedFlow[i] == 0 || FlowRate[i] == 0)\n        {\n           ; /* nothing */\n        }\n        else if (Drawing[i] == 1)          /* anchor found */\n        {\n            EventIndex = i;                /* provisional */\n\n            /* back-fill earlier low-flow purging samples      */\n            for (j = i - 1; j >= 0; j--)\n            {\n                if (Purging[j] == 1 &&\n                    TotalizedFlow[j] >  0.0 &&\n                    TotalizedFlow[j] <= 0.5)\n                {\n                    EventIndex = j;        /* shift anchor   */\n                }\n                else\n                {\n                    break;                 /* stop back-fill */\n                }\n            }\n            break;                         /* anchor secured */\n        }\n    }\n}\n/* ===== any other Index_Type ? EventIndex remains -1 ============== */"() -> ()  [unwired: 7 in, 1 out]
    }
    frame Enabled {
    }
  }
  n39 = Array Size(array=w12) -> (size(s)=w17:i32)
  n40 = To Long Integer(number=w12) -> (32bit integer=w14:i32[])
  n41 = formula code="/*********************************************************************\n *  FIND FIRST “ACTIVE” SAMPLE (EventIndex)                          *\n *                                                                   *\n *  Index_Type (scalar)                                              *\n *    1 ? Heating: first sample where Heat_Source ? 0                *\n *              (expressed with “== 0” logic, no “!=”)               *\n *    0 ? Drawing / Purging:                                         *\n *        • Locate first Drawing == 1                                *\n *        • Walk backward to include any earlier low-flow Purging    *\n *        • If no Drawing exists, EventIndex stays -1                *\n *                                                                   *\n *  OUTPUT : int32  EventIndex   (-1 ? “no qualifying sample”)       *\n *                                                                   *\n *  STYLE NOTES                                                      *\n *    • No “!=” comparisons—only “== 0” plus else branches           *\n *    • No “continue”; flow is linear                                *\n *    • A single break exits a loop once the answer is found         *\n *********************************************************************/\n\n/* -------- Inputs (all arrays length N) --------------------------- */\nint32 i, j;    // These are the index counters\nint32 curDrawCnt;\n\n/*------------------------------------------------------------------*/\n\nint32 EventIndex = -1;    /* default: nothing found */\n\n/* ========================== HEATING ============================== */\nif (Index_Type == 1)\n{\n    for (i = 0; i < N; i++)\n    {\n        /* Heater off , keep searching; Heater on, record & exit */\n        if (Heat_Source[i] == 0)\n        {\n            ; // still off\n        }\n        else if (Heat_Source[i] == 1)                      // heater on\n        {\n            EventIndex = StartIndex+i;\n            break;                 // done\n        }\n    }\n}\n\n/* ==================== DRAWING / PURGING ========================= */\nelse if (Index_Type == 0)\n{\n    for (i = 0; i < N; i++)\n    {\n        /* ---------- 0) per-row flags --------------------------- */\n        int32 validFlow   = 0;   /* default FALSE  */\n        int32 drawCountOK = 1;   /* default PASS   */\n\n        /* ---------- 1)  VALID-FLOW test ------------------------ */\n        if (TotalizedFlow[i] > 0.0)                    /* volume seen  */\n        {\n            /* A) totalizer climbed since previous sample           */\n            if (i > 0 && TotalizedFlow[i] > TotalizedFlow[i - 1])\n            {\n                validFlow = 1;\n            }\n            /* B) FlowRate positive with a non-zero neighbour       */\n            else if (FlowRate[i] > 0.0)\n            {\n                int32 prevNonZero = 0;\n                int32 nextNonZero = 0;\n\n                if (i > 0)\n                    prevNonZero = (FlowRate[i - 1] == 0.0) ? 0 : 1;\n\n                if (i < N - 1)\n                    nextNonZero = (FlowRate[i + 1] == 0.0) ? 0 : 1;\n\n                if (prevNonZero == 1 || nextNonZero == 1)\n                    validFlow = 1;\n            }\n        }\n\n        /* ---------- 2)  Extra draw-count filter ---------------- */\n        /* The new Draw_Count should be different than Draw_Count_Start, if its the same, there is an error that you should skip */\n        if (Loop_Index > 0)\n        {\n            curDrawCnt = Draw_Count[i];\n            if (curDrawCnt == Draw_Count_Start)        /* counter flat */\n                drawCountOK = 0;                       /* skip sample  */\n        }\n\n        /* ---------- 3)  Drawing anchor check ------------------- */\n        if (validFlow == 1 && Drawing[i] == 1 && drawCountOK == 1)\n        {\n            EventIndex = StartIndex + i;               /* anchor       */\n\n            /* ---- back-fill earlier low-flow Purging ------------ */\n            for (j = i - 1; j >= 0; j--)\n            {\n                if (Purging[j] == 1 &&\n                    TotalizedFlow[j] > 0.0 &&\n                    TotalizedFlow[j] <= 0.5)\n                {\n                    EventIndex = StartIndex + j;       /* shift back   */\n                }\n                else\n                {\n                    break;                             /* exit zone    */\n                }\n            }\n            break;                                     /* anchor done  */\n        }\n        /* else: keep scanning for next i */\n    }\n}\n/* ===== any other Index_Type – EventIndex remains -1 ============ */"("TotalizedFlow"=w24, "FlowRate"=w20, "Drawing"=w29, "Purging"=w30, "Index_Type"="Index Type", "Heat_Source"=w14, "N"=w17, "StartIndex"=w8, "Loop_Index"="Loop Index", "Draw_Count"=w6, "Draw_Count_Start"=w1) -> ("EventIndex"=w11:i32)
  "Draw Start" <- w11
  n42 = Equal?(x=w11, y=-1) -> (x = y?=→"Stop Searching":bool)
  "Error Out" <- "Error In"
  "UEF Calculated Values Output" <- "UEF Calculated Values in"
